vi "worksheet set zoom.vi"(8 "error in (no error)":errorcluster, 10 "scale":u16, 11 "worksheet":u32) -> (0 "error out":errorcluster)   [LabVIEW 2015, in "xlsxwriter.lvlib"]
doc: "void worksheet_set_zoom(lxw_worksheet worksheet, uint16_t scale);"
uses:
  xlsxwriter.lvlib
  xlsxwriter.dll
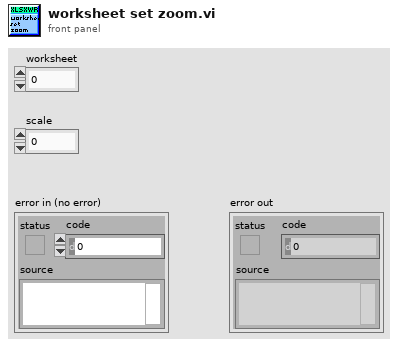
[diagram p1: front panel]
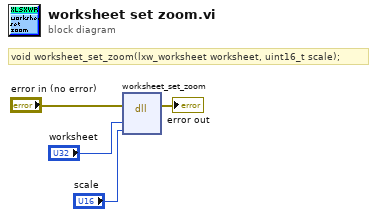
[diagram p0: block diagram]
diagram:
  # "void worksheet_set_zoom(lxw_worksheet worksheet, uint16_t scale);"
  n1 = dll-call lib="C:/Users/WDAGUtilityAccount/Desktop/lv_vis_added_cell/xlsxwriter.*" fn="worksheet_set_zoom"(error in="error in (no error)", "worksheet"="worksheet", "scale"="scale") -> (error out=→"error out":errorcluster)  [unwired: 5 in, 1 out]
